vi "LIMITXdll.vi"(8 "error in (no error)":errorcluster, 11 "Inputs":T2) -> (0 "error out":errorcluster, 3 "Outputs":T1)   [LabVIEW 2015]
doc: "subroutine LIMITXdll(htyp, t, d, p, z, tmin, tmax, dmax, pmax, ierr, herr, htyp_length, herr_length)\n\nReturns limits of a property model as a function of composition and/or checks inputs T, D, and P against those\nlimits.\n\nPure fluid limits are read in from the *.fld files; for mixtures, a simple mole fraction weighting of the reduced\nvariables is used.\n\nAttempting calculations below the minimum temperature and/or above the maximum density may result in an\nerror. These will often correspond to a physically unreasonable state; also many equations of state do not\nextrapolate reliably to lower T’s and higher D’s.\n\nA warning is issued if the temperature is above the maximum but below 1.5 times the maximum. Pressures up\nto twice the maximum result in only a warning. Most equations of state may be extrapolated to higher T’s and\nP’s. Temperatures and/or pressures outside these extended limits will result in an error.\n\nWhen calling with an unknown temperature, set T to -1 to avoid performing the melting line check. If inputs are\nnot available, use T=300, P=0, and D=0.\n\nIf multiple inputs are outside limits, ierr=SUM(ABS(ierr)), with a positive sign if any error greater than zero\n(calculations not possible), or a negative sign for warnings only.\n\nINPUTS:\nhtyp -- Flag indicating the model to check (character*3)\n ‘EOS’: Equation of state\n ‘ETA’: Viscosity \n ‘TCX’: Thermal conductivity \n ‘STN’: Surface tension\nt -- Temperature [K]\nD -- Molar density [mol/L]\np -- Pressure [kPa]\nz -- Composition array (array of mole fractions)\n\nOUTPUTS:\ntmin -- Minimum temperature for model specified by htyp [K]\ntmax -- Maximum temperature [K]\ndmax -- Maximum density [mol/L]\npmax -- Maximum pressure [kPa]\nierr -- Error flag:\n 0 = All inputs within limits\n -1 = 1.5*Tmax > T > Tmax\n 1 = T < Tmin or T > 1.5*Tmax\n 2 = D > Dmax or D < 0\n -4 = 2*Pmax > P > Pmax\n 4 = P < 0 or P > 2*Pmax\n 8 = Component composition < 0 or > 1 and/or composition sum <> 1\n 16 = P>Pmelt\n -16 = T<Ttrp (important for water)\nherr -- Error string (character*255)\nhtyp_length -- length of variable htyp (default: 3)\nherr_length -- length of variable herr (default: 255)"
uses:
  REFPROP.dll
panel:
  # "REFPROP-LIMITXdll.vi"
  # "void  LIMITXdll(CStr htyp, double *t, double *D, double *p, double *z, double *tmin, double *tmax, double *dmax, double *pmax, int32_t *ierr, CStr herr, int32_t htyp_length, int32_t herr_length)"
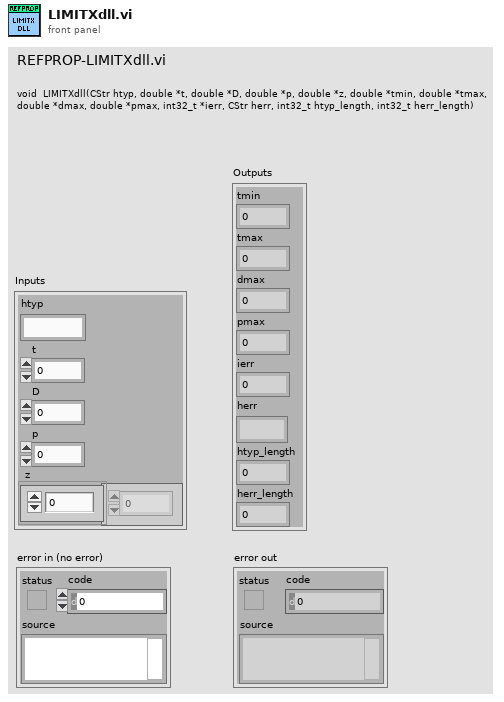
[diagram p1: front panel]
types:
  T1 = cluster{"tmin":dbl, "tmax":dbl, "dmax":dbl, "pmax":dbl, "ierr":i32, "herr":string, "htyp_length":i32, "herr_length":i32}
  T2 = cluster{"htyp":string, "t":dbl, "D":dbl, "p":dbl, "z":dbl[]}
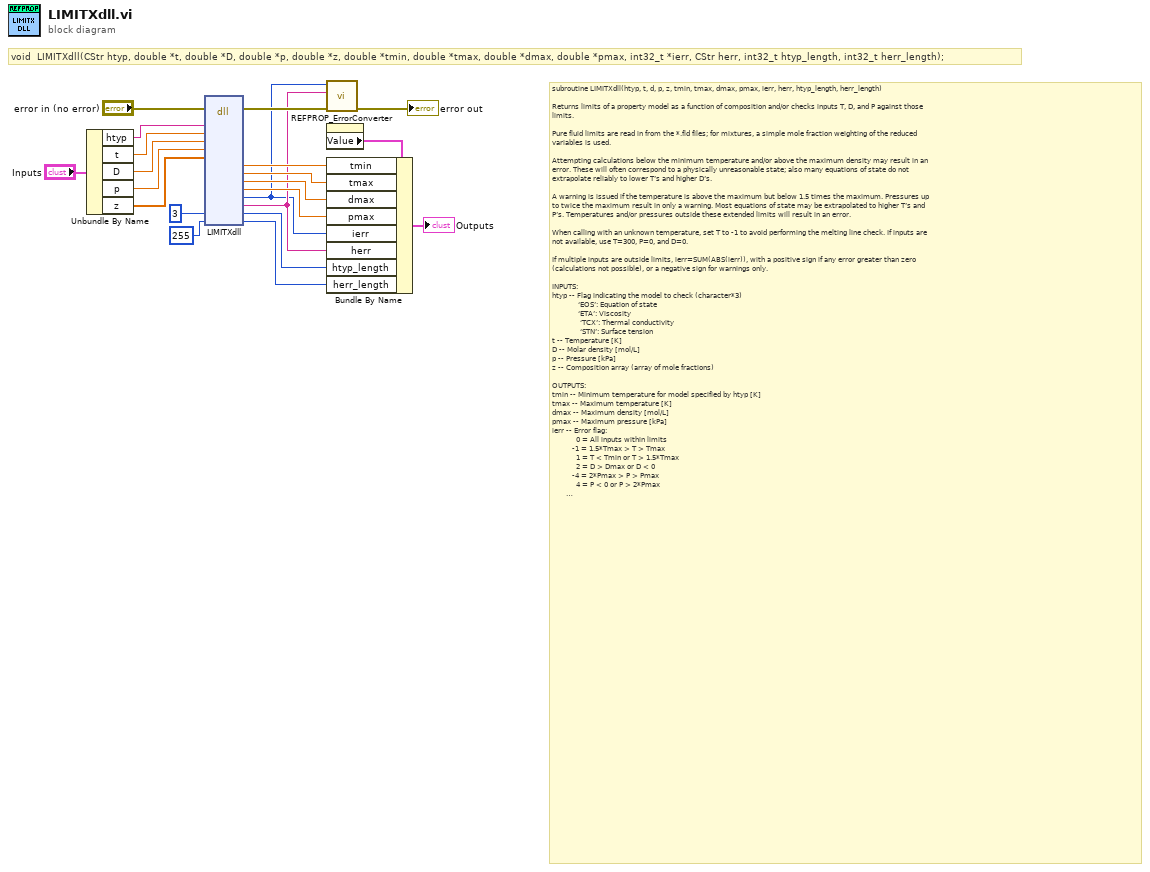
[diagram p0: block diagram]
diagram:
  # "void  LIMITXdll(CStr htyp, double *t, double *D, double *p, double *z, double *tmin, double *tmax, double *dmax, double *pmax, int32_t *ierr, CStr herr, int32_t htyp_length, int32_t herr_length);"
  # "subroutine LIMITXdll(htyp, t, d, p, z, tmin, tmax, dmax, pmax, ierr, herr, htyp_length, herr_length)\n\nReturns limits of a property model as a function of composition and/or checks inputs T, D, and P against those\nlimits.\n\nPure fluid limits are read in from the *.fld files; for mixtures, a simple mole fraction weighting of the reduced\nvariables is used.\n\nAttempting calculations below the minimum temperature and/or above the maximum density may result in an\nerror. These will often correspond to a physically unreasonable state; also many equations of state do not\nextrapolate reliably to lower T’s and higher D’s.\n\nA warning is issued if the temperature is above the maximum but below 1.5 times the maximum. Pressures up\nto twice the maximum result in only a warning. Most equations of state may be extrapolated to higher T’s and\nP’s. Temperatures and/or pressures outside these extended limits will result in an error.\n\nWhen calling with an unknown temperature, set T to -1 to avoid performing the melting line check. If inputs are\nnot available, use T=300, P=0, and D=0.\n\nIf multiple inputs are outside limits, ierr=SUM(ABS(ierr)), with a positive sign if any error greater than zero\n(calculations not possible), or a negative sign for warnings only.\n\nINPUTS:\nhtyp -- Flag indicating the model to check (character*3)\n             ‘EOS’: Equation of state\n             ‘ETA’: Viscosity \n              ‘TCX’: Thermal conductivity \n              ‘STN’: Surface tension\nt -- Temperature [K]\nD -- Molar density [mol/L]\np -- Pressure [kPa]\nz -- Composition array (array of mole fractions)\n\nOUTPUTS:\ntmin -- Minimum temperature for model specified by htyp [K]\ntmax -- Maximum temperature [K]\ndmax -- Maximum density [mol/L]\npmax -- Maximum pressure [kPa]\nierr -- Error flag:\n            0 = All inputs within limits\n          -1 = 1.5*Tmax > T > Tmax\n            1 = T < Tmin or T > 1.5*Tmax\n            2 = D > Dmax or D < 0\n          -4 = 2*Pmax > P > Pmax\n            4 = P < 0 or P > 2*Pmax\n            8 = Component composition < 0 or > 1 and/or composition sum <> 1\n            16 = P>Pmelt\n          -16 = T<Ttrp (important for water)\nherr -- Error string (character*255)\nhtyp_length -- length of variable htyp (default: 3)\nherr_length -- length of variable herr (default: 255)"
  n1 = Unbundle By Name("Inputs") -> ("htyp"=w15:string, "t"=w14:dbl, "D"=w13:dbl, "p"=w12:dbl, "z"=w11:dbl[])
  n2 = dll-call lib="C:/Users/lauria/Desktop/REFPROP 10 LabVIEW Wrapper BETA/REFPROP/REFPROP.*" fn="LIMITXdll"(error in="error in (no error)", "htyp"=w15, "t"=w14, "D"=w13, "p"=w12, "z"=w11, "htyp_length"=3 ("ln1"), "herr_length"=255 ("ln2")) -> (error out=w19:errorcluster, "tmin"=w8:dbl, "tmax"=w7:dbl, "dmax"=w6:dbl, "pmax"=w5:dbl, "ierr"=w1:i32, "herr"=w2:string, "htyp_length"=w3:i32, "herr_length"=w4:i32)  [unwired: 14 in, 1 out]
  n3 = call "REFPROP_ErrorConverter.vi"("error in (no error)"=w19, "Error Message"=w2, "Error Code"=w1) -> ("error out"=→"error out":errorcluster)  [unwired: 8 in]
  n4 = property on="Outputs" class="Clust (strict)"() -> ("Value"=w9:T1)  [unwired: 2 in, 2 out]
  n5 = Bundle By Name(cluster=w9, "tmin"=w8, "tmax"=w7, "dmax"=w6, "pmax"=w5, "ierr"=w1, "herr"=w2, "htyp_length"=w3, "herr_length"=w4) -> (→"Outputs":T1)
